vi "6-3 웹브라우저.vi"() -> ()   [LabVIEW 2014]
panel:
  out "에러 출력":errorcluster
  in  "WebBrowser":refnum<k7>(container)
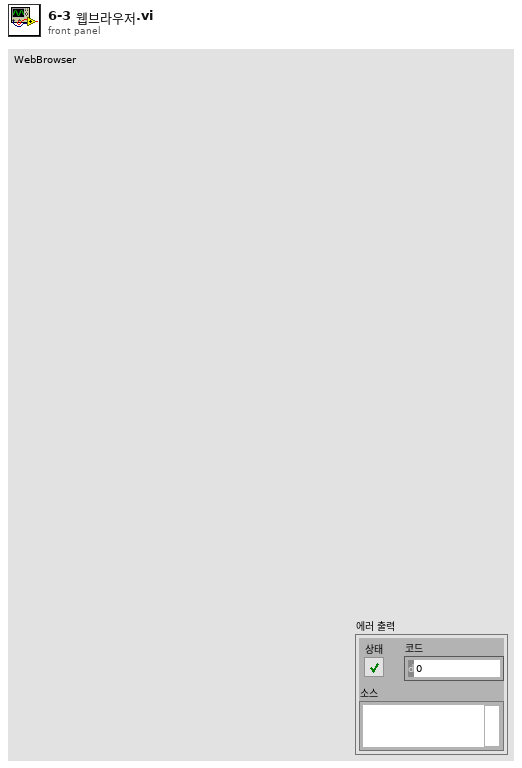
[diagram p1: front panel]
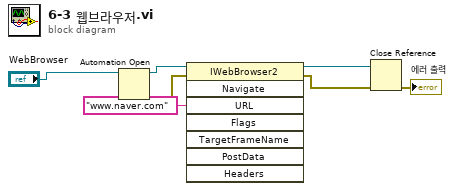
[diagram p0: block diagram]
diagram:
  n1 = Automation Open(Automation Refnum="WebBrowser") -> (Automation Refnum=w6:refnum<k7>, error out=w4:errorcluster)  [unwired: 3 in]
  n2 = invoke class="IWebBrowser2" method="Navigate"(reference=w6, error in=w4, "URL"="www.naver.com") -> (reference out=w5:refnum<k7>, error out=w3:errorcluster)  [unwired: 5 in, 6 out]
  n3 = Close Reference(reference=w5, error in (no error)=w3) -> (error out=→"에러 출력":errorcluster)
